vi "Shutdown.vi"(8 "Error In":errorcluster, 11 "SSH":refnum<class "SSH.lvclass">) -> (0 "Error Out":errorcluster)   [LabVIEW 2018, in "Toolkit.lvlib" / "SSH.lvclass"]
doc: "Cleanly and safely shutdowns the underlying libssh2 shared library. This must be called, or executed, after all other VI within this toolkit are completed. Once this is called, no other VIs from this toolkit should be called, or executed. This frees all internal memory used by the libssh2 shared library and a segmentation fault will occur if toolkit VIs are executed after this VI is executed."
uses:
  SSH.lvclass
  SSH.lvclass/SSH.ctl
  Toolkit.lvlib
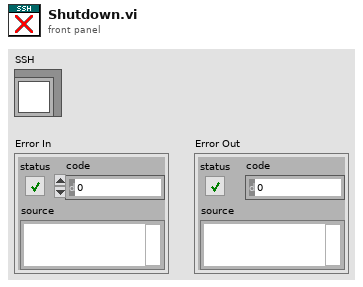
[diagram p1: front panel]
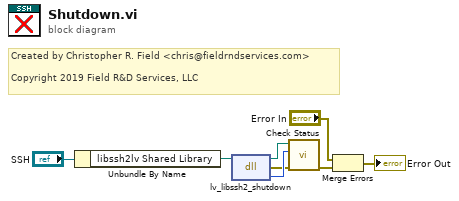
[diagram p0: block diagram]
diagram:
  # "Created by Christopher R. Field <chris@fieldrndservices.com>\n\nCopyright 2019 Field R&D Services, LLC"
  n1 = Unbundle By Name("SSH") -> ("libssh2lv Shared Library"=w2:path)
  n2 = dll-call lib="D:/Users/cfield/Code/Field R&D Services/SSH/LV-LIBSSH2/LabVIEW/trunk/src/Toolkit/Support/lv-libssh2.*" fn="lv_libssh2_shutdown"(path in=w2) -> (path out=w6:path, error out=w4:errorcluster, "return type"=w5:i32)  [unwired: 2 in]
  n3 = call "Check Status.vi"("Error In"=w4, "Status"=w5, "lv-libssh2 Shared Library In"=w6) -> ("Error Out"=w1:errorcluster)  [unwired: 7 in, 1 out]
  n4 = Merge Errors("Error In", w1) -> (→"Error Out":errorcluster)
